vi "SetInputChannels_SubVI.vi"(8 "Channels":T1[](array[typedef]) {"DeadTime" min=800 max=160000 step=1; "Edge" items=["falling", "rising"]; "Offset" min=-100000 max=100000 step=10; "Level" min=-1200 max=1200 step=1}, 9 "SetInpChan":T2[](array[typedef]), 10 "features":i32, 11 "DevIdx":i32) -> (0 "error out":errorcluster)   [LabVIEW 2023]
uses:
  Types/MH_SetInpChanData.ctl
  Types/MH_SetInpChanCmds.ctl
  Types/MH_InputChannel.ctl
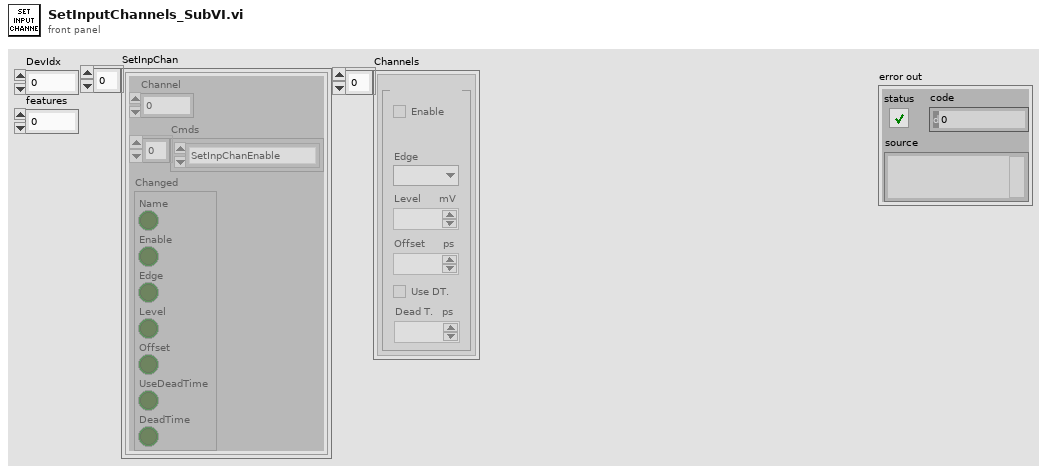
[diagram p1: front panel]
types:
  T1 = typedef "MH_InputChannel.ctl" = cluster{"Name":string, "Enable":bool, "Edge":i32, "Level":i32, "Offset":i32, "UseDeadTime":bool, "DeadTime":i32}
  T2 = typedef "MH_SetInpChanData.ctl" = cluster{"Channel":i32, "Cmds":T3[], "Changed":cluster{"Name":bool, "Enable":bool, "Edge":bool, "Level":bool, "Offset":bool, "UseDeadTime":bool, "DeadTime":bool}}
  T3 = typedef "MH_SetInpChanCmds.ctl" = enum16{"SetInpChanEnable", "SetInpChanOffset", "SetInpChanDeadTime", "SetInpChanTrg"}
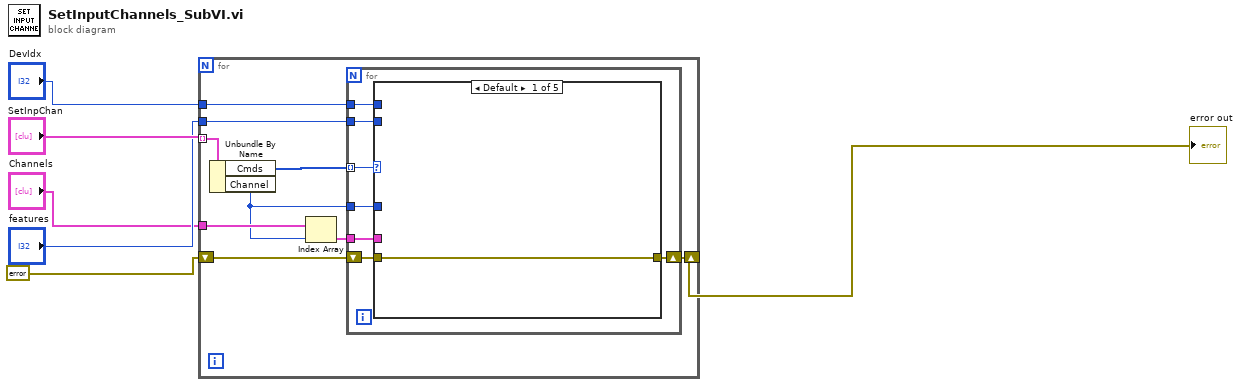
[diagram p0: block diagram]
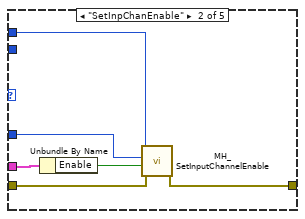
[diagram p2: hidden frame]
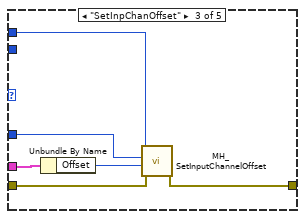
[diagram p3: hidden frame]
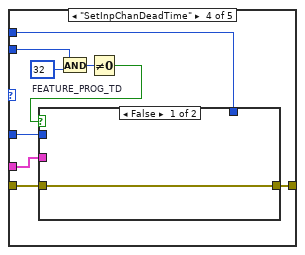
[diagram p4: hidden frame]
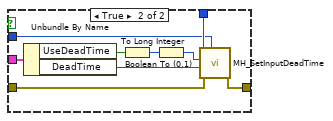
[diagram p5: hidden frame]
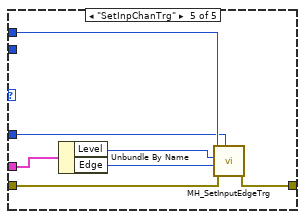
[diagram p6: hidden frame]
diagram:
  n1 = for {
    tunnel: "Channels" -> [w11]
    tunnel: "SetInpChan" -> [w15] mode=indexing
    shift-right: [w13] -> w5
    shift-left: errorcluster {"status"=FALSE, "code"=0, "source"=""} ("error out") -> [w12]
    tunnel: "DevIdx" -> [w9]
    tunnel: "features" -> [w7]
    n2 = Unbundle By Name(w15) -> ("Cmds"=w14:T3[], "Channel"=w8:i32)
    n3 = Index Array(array=w11, index=w8) -> (element=w10:T1)
    n4 = for {
      tunnel: w14 -> [w22] mode=indexing
      tunnel: w8 -> [w21]
      shift-right: [w20] -> w13
      shift-left: w12 -> [w19]
      tunnel: w10 -> [w18]
      tunnel: w9 -> [w17]
      tunnel: w7 -> [w16]
      n5 = case shown="Default" w22 {
        tunnel: w21 -> [_ w28 w35 w40 w56]
        tunnel: [w23 w27 w34 w44 w61] -> w20
        tunnel: w19 -> [w23 w26 w33 w43 w60]
        tunnel: w18 -> [_ w25 w32 w42 w59]
        tunnel: w17 -> [_ w24 w31 w41 w58]
        tunnel: w16 -> [_ _ _ w37 _]
        frame Default {
        }
        frame "SetInpChanEnable" {
          n6 = Unbundle By Name(w25) -> ("Enable"=w29:bool)
          n7 = call "MH_SetInputChannelEnable.vi"("error in (no error)"=w26, "enable"=w29, "channel"=w28, "devidx"=w24) -> ("error out"=w27:errorcluster)  [unwired: 6 in, 1 out]
        }
        frame "SetInpChanOffset" {
          n8 = Unbundle By Name(w32) -> ("Offset"=w30:i32)
          n9 = call "MH_SetInputChannelOffset.vi"("error in (no error)"=w33, "Offset"=w30, "channel"=w35, "devidx"=w31) -> ("error out"=w34:errorcluster)  [unwired: 6 in, 1 out]
        }
        frame "SetInpChanDeadTime" {
          w38 = 32  # FEATURE_PROG_TD
          n10 = And(x=w37, y=w38) -> (x .and. y?=w39:i32)
          n11 = Not Equal To 0?(x=w39) -> (x != 0?=w36:bool)
          n12 = case shown="False" w36 {
            tunnel: [w45 w54] -> w44
            tunnel: w43 -> [w45 w53]
            tunnel: w42 -> [_ w52]
            tunnel: w41 -> [_ w51]
            tunnel: w40 -> [_ w49]
            frame False {
            }
            frame True {
              n13 = Unbundle By Name(w52) -> ("UseDeadTime"=w48:bool, "DeadTime"=w50:i32)
              n14 = Boolean To (0,1)(Boolean=w48) -> (0, 1=w47:i16)
              n15 = To Long Integer(number=w47) -> (32bit integer=w46:i32)
              n16 = call "MH_SetInputDeadTime.vi"("channel"=w49, "error in (no error)"=w53, "deadtime"=w50, "on"=w46, "devidx"=w51) -> ("error out"=w54:errorcluster)  [unwired: 5 in, 1 out]
            }
          }
        }
        frame "SetInpChanTrg" {
          n17 = Unbundle By Name(w59) -> ("Level"=w55:i32, "Edge"=w57:i32)
          n18 = call "MH_SetInputEdgeTrg.vi"("channel"=w56, "error in (no error)"=w60, "edge"=w57, "level"=w55, "devidx"=w58) -> ("error out"=w61:errorcluster)  [unwired: 5 in, 1 out]
        }
      }
    }
  }
  "error out" <- w5
